vi "Type to colour String.vi"(11 "Type":string) -> (3 "Requested Colour":T1)   [LabVIEW 2018]
doc: "Identifies the correct colour string to use for each supported data type (blue for integers, orange for floating point numbers, pink for strings and green for booleans)"
uses:
  Icon Colours.ctl
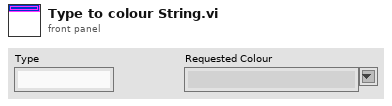
[diagram p1: front panel]
types:
  T1 = typedef "Icon Colours.ctl" = string
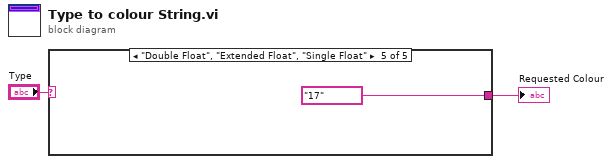
[diagram p0: block diagram]
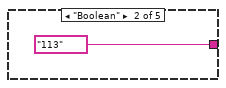
[diagram p3: hidden frame]
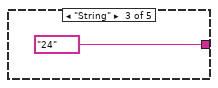
[diagram p4: hidden frame]
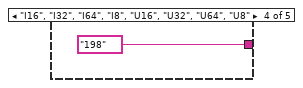
[diagram p5: hidden frame]
diagram:
  n1 = case shown="\"Double Float\", \"Extended Float\", \"Single Float\"" "Type" {
    tunnel: [_ T1 "113" ("Requested Colour") T1 "24" ("Requested Colour") T1 "198" ("Requested Colour") T1 "17" ("Requested Colour")] -> w2
    frame Default {
    }
    frame "Boolean" {
    }
    frame "String" {
    }
    frame "I16", "I32", "I64", "I8", "U16", "U32", "U64", "U8" {
    }
    frame "Double Float", "Extended Float", "Single Float" {
    }
  }
  "Requested Colour" <- w2
